vi "Add Line.vi"(8 "error in":errorcluster, 10 "String":string, 11 "Console Log in":refnum<class "Console Log.lvclass">) -> (0 "error out":errorcluster, 3 "Console Log out":refnum<class "Console Log.lvclass">)   [LabVIEW 2011, in "Console Log.lvclass"]
uses:
  Console Log.lvclass
  Console Log.lvclass/Console Log.ctl
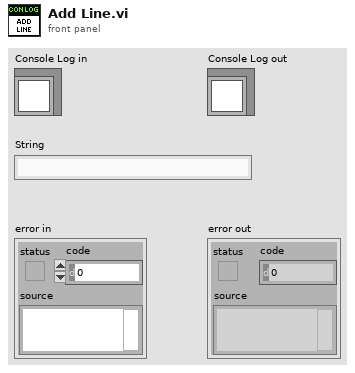
[diagram p1: front panel]
types:
  T1 = enum16{"open", "replace", "create", "open or create", "replace or create", "replace or create with confirmation"}
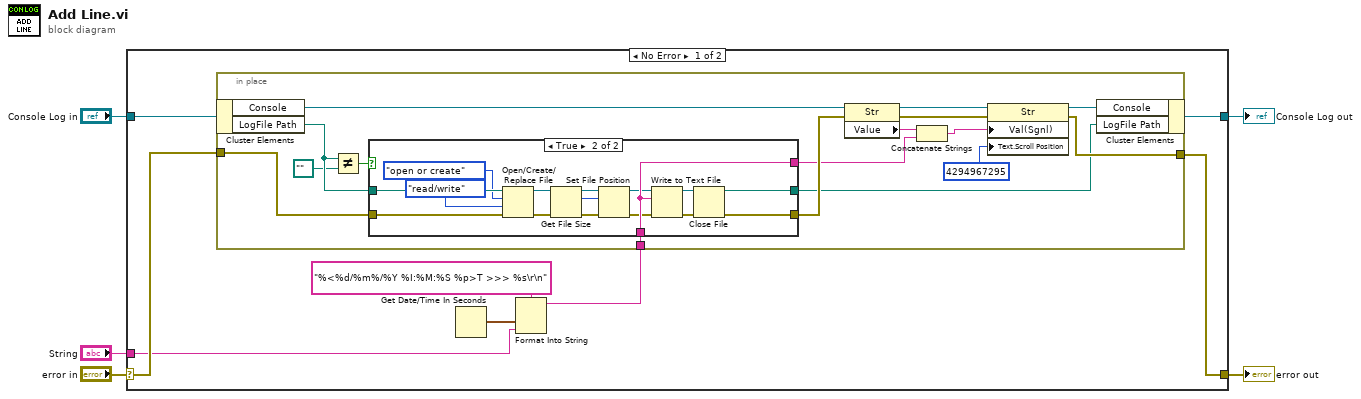
[diagram p0: block diagram]
diagram:
  n1 = case shown="No Error" "error in" {
    selector: "error in" -> [w11 w50]
    tunnel: [w10 w50] -> w4
    tunnel: [w12 w49] -> w2
    tunnel: "Console Log in" -> [w13 w49]
    tunnel: "String" -> [w8 _]
    frame No Error {
      n2 = Get Date/Time In Seconds() -> (seconds since 1Jan1904=w6:timestamp)
      n3 = Format Into String(format string="%<%d/%m%/%Y %I:%M:%S %p>T >>> %s\r\n", w6, w8) -> (resulting string=w7:string)  [unwired: 2 in, 1 out]
      n4 = in-place {
        in-place-border: w11 -> [w21]
        in-place-border: [w24] -> w10
        in-place-border: w7 -> [w20]
        n5 = in-place-cluster #1(w13) -> ("Console"=w29:refnum<vi>, "LogFile Path"=w17:path)
        n6 = Not Equal?(x=w17, y=path "") -> (x != y?=w15:bool)
        n7 = case shown="True" w15 {
          tunnel: w17 -> [w32 w48]
          tunnel: w21 -> [w31 w45]
          tunnel: w20 -> [w30 w40]
          tunnel: [w31 w42] -> w19
          tunnel: [w32 w41] -> w18
          tunnel: [w30 w40] -> w14
          frame False {
          }
          frame True {
            n8 = Open/Create/Replace File(file path (use dialog)=w48, error in=w45, operation (0:open)=T1."open or create", access (0:read/write)=enum16{"read/write", "read-only", "write-only"}."read/write") -> (refnum out=w38:refnum<file>, error out=w36:errorcluster)  [unwired: 2 in, 1 out]
            n9 = Get File Size(file=w38, error in=w36) -> (refnum out=w37:refnum<file>, size (in bytes)=w39:i64, 0:w35:errorcluster)
            n10 = Set File Position(offset (in bytes) (0)=w39, refnum=w37, error in=w35) -> (refnum out=w34:refnum<file>, error out=w33:errorcluster)  [unwired: 1 in]
            n11 = Write to Text File(file (use dialog)=w34, text=w40, error in=w33) -> (refnum out=w43:refnum<file>, error out=w44:errorcluster)  [unwired: 1 in, 1 out]
            n12 = Close File(refnum=w43, error in=w44) -> (path=w41:path, error out=w42:errorcluster)
          }
        }
        n13 = property class="Str"(reference=w29, error in=w19) -> (reference out=w27:refnum<vi>, error out=w28:errorcluster, "Value"=w23:string)
        n14 = Concatenate Strings(w23, w14) -> (w26:string)
        n15 = property class="Str"(reference=w27, error in=w28, "Val(Sgnl)"=w26, "Text.Scroll Position"=u32 4294967295) -> (reference out=w25:refnum<vi>, error out=w24:errorcluster)
        n16 = in-place-cluster #1("Console"=w25, "LogFile Path"=w18) -> (w12:refnum<class "Console Log.lvclass">)
      }
    }
    frame Error {
    }
  }
  "error out" <- w4
  "Console Log out" <- w2
